vi "Fluence in Area.vi"(0 "Masked Image (I16only)":T2, 1 "Origin Image":i64[][](array[numeric]), 5 "Energie":dbl[unit], 7 "calibration mm/px":dbl[unit], 9 "Size of region":i32, 11 "error in (no error)":errorcluster) -> (6 "Fluence J/cm^2":dbl[unit], 8 "Energy in Area":dbl[unit], 10 "Max fluence area":T1, 14 "max value":i64, 15 "error out":errorcluster)   [LabVIEW 2014, in "Analyze.lvlib" / "Analyze Fluence.lvclass"]
uses:
  Analyze Fluence.lvclass
  <vilib>/vision/Image Controls.llb/IMAQ Image.ctl
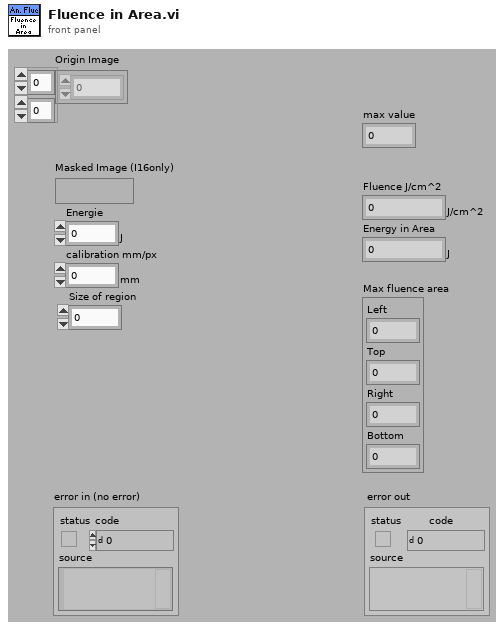
[diagram p1: front panel]
types:
  T1 = cluster{"Left":i32, "Top":i32, "Right":i32, "Bottom":i32}
  T2 = typedef "IMAQ Image.ctl" = refnum<image>
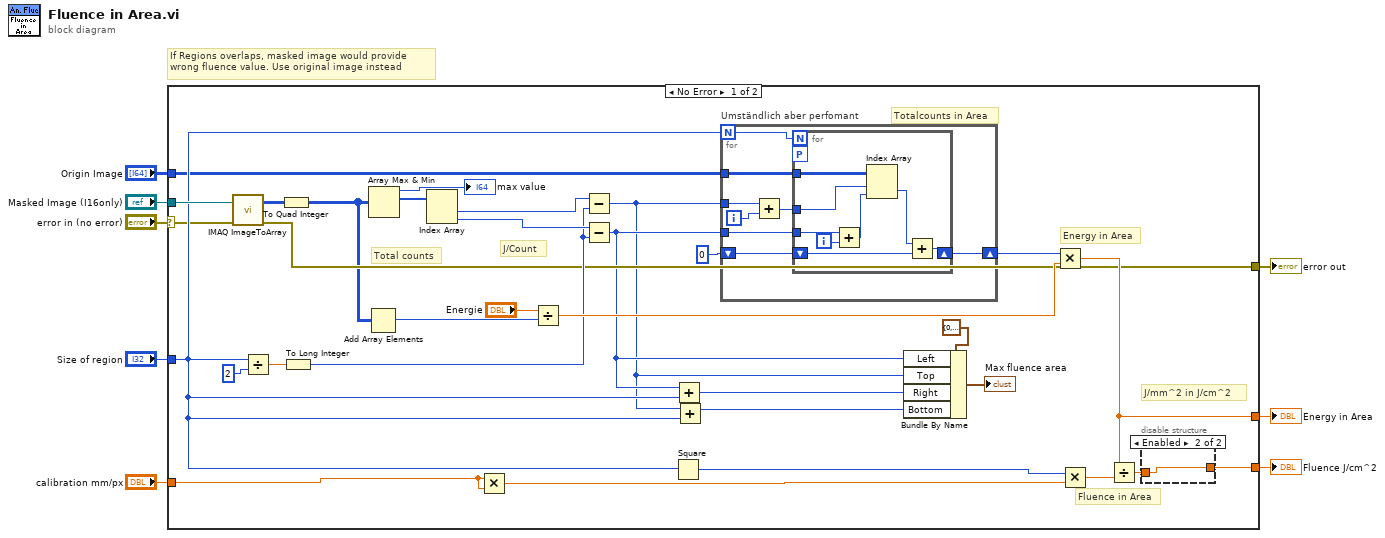
[diagram p0: block diagram]
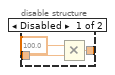
[diagram p2: hidden frame]
diagram:
  # "If Regions overlaps, masked image would provide \nwrong fluence value. Use original image instead"
  n1 = case shown="No Error" "error in (no error)" {
    selector: "error in (no error)" -> [w9 w61]
    tunnel: [w27 _] -> w8
    tunnel: [w22 _] -> w7
    tunnel: "Masked Image (I16only)" -> [w21 _]
    tunnel: [w20 w61] -> w5
    tunnel: "Size of region" -> [w14 _]
    tunnel: "Origin Image" -> [w12 _]
    tunnel: "calibration mm/px" -> [w10 _]
    frame No Error {
      # "J/mm^2 in J/cm^2"
      # "Fluence in Area"
      # "Totalcounts in Area"
      # "Energy in Area"
      # "J/Count"
      # "Total counts"
      n2 = call "IMAQ ImageToArray"("error in (no error)"=w9, "Image"=w21) -> ("error out"=w20:errorcluster, "Image Pixels (I16)"=w18:i16[][])  [unwired: 2 in, 3 out]
      n3 = Divide(x=w14, y=u16 2) -> (x/y=w36:dbl)
      n4 = To Quad Integer(1:w18) -> (0:w17:i64[][])
      n5 = To Long Integer(number=w36) -> (32bit integer=w28:i32)
      n6 = Add Array Elements(numeric array=w17) -> (sum=w26:i64)
      n7 = Array Max & Min(array=w17) -> (max value=→"max value":i64, max index (indices)=w40:i32[])  [unwired: 2 out]
      n8 = Index Array(array=w40) -> (element #1=w37:i32, element #2=w35:i32)  [unwired: 2 in]
      n9 = Multiply(x=w10, y=w10) -> (x*y=w33:dbl[unit])
      n10 = Divide(x="Energie", y=w26) -> (x/y=w34:dbl[unit])
      n11 = Subtract(x=w37, y=w28) -> (x-y=w11:i32)
      n12 = Subtract(x=w35, y=w28) -> (x-y=w16:i32)
      n13 = Square(x=w14) -> (x^2=w32:i32)
      n14 = Add(x=w16, y=w14) -> (x+y=w24:i32)
      n15 = Add(x=w11, y=w14) -> (x+y=w25:i32)
      n16 = for "Umständlich aber perfomant" {
        N: w14 -> [w45]
        tunnel: w11 -> [w51]
        tunnel: w16 -> [w52]
        shift-right: [w49] -> w13
        shift-left: i64 0 -> [w50]
        tunnel: w12 -> [w48]
        i -> [w46]
        n17 = Add(x=w51, y=w46) -> (x+y=w47:i32)
        n18 = for {
          N: w45 -> [_]
          tunnel: w52 -> [w56]
          tunnel: w47 -> [w60]
          shift-right: [w54] -> w49
          shift-left: w50 -> [w59]
          tunnel: w48 -> [w58]
          workers-P: _ -> [_]
          i -> [w57]
          n19 = Add(x=w56, y=w57) -> (x+y=w55:i32)
          n20 = Index Array(array=w58, index (row)=w60, index (col)=w55) -> (element=w53:i64)
          n21 = Add(x=w53, y=w59) -> (x+y=w54:i64)
        }
      }
      n22 = Bundle By Name(cluster=T1 {"Left"=0, "Top"=0, "Right"=0, "Bottom"=0} ("Rectangle"), "Left"=w16, "Top"=w11, "Right"=w24, "Bottom"=w25) -> (→"Max fluence area":T1)
      n23 = Multiply(x=w13, y=w34) -> (x*y=w27:dbl[unit])
      n24 = Multiply(x=w32, y=w33) -> (x*y=w31:dbl[unit])
      n25 = Divide(x=w27, y=w31) -> (x/y=w23:dbl[unit])
      n26 = disable-structure shown="Enabled" {
        disable-tunnel: w23 -> [w43 w44]
        disable-tunnel: [w42 w44] -> w22
        frame Disabled {
          n27 = Multiply(x=100.0, y=w43) -> (x*y=w42:dbl[unit])
        }
        frame Enabled {
        }
      }
    }
    frame Error {
    }
  }
  "Fluence J/cm^2" <- w7
  "Energy in Area" <- w8
  "error out" <- w5
